vi "TDMS Timestamp and Data Double.vi"(6 "channel name(s) in (Untitled)":string[](array[string]), 7 "timestamp":timestamp, 8 "error in (no error)":errorcluster, 9 "group name in (Untitled)":string, 10 "Array":dbl[](array[numeric]), 11 "Refnum in":refnum<k34>) -> (0 "error out":errorcluster, 3 "Refnum out":refnum<k34>)   [LabVIEW 2014]
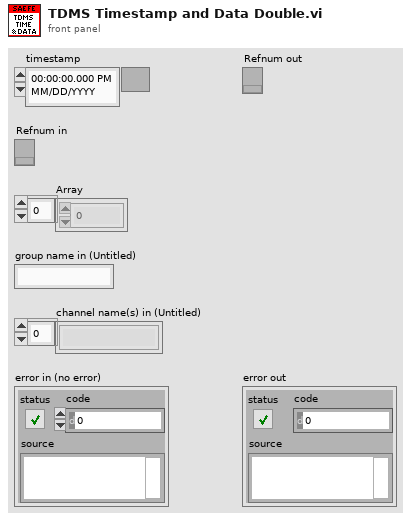
[diagram p1: front panel]
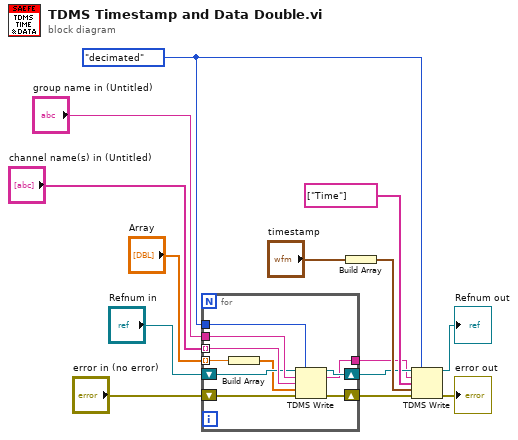
[diagram p0: block diagram]
diagram:
  w12 = enum16{"decimated", "interleaved"}."decimated" ("data layout (0:decimated)")
  n1 = for {
    tunnel: w12 -> [w24]
    tunnel: "Array" -> [w17] mode=indexing
    tunnel: "channel name(s) in (Untitled)" -> [w21] mode=indexing
    tunnel: "group name in (Untitled)" -> [w20]
    shift-right: [w23] -> w7
    shift-left: "error in (no error)" -> [w19]
    shift-right: [w22] -> w6
    shift-left: "Refnum in" -> [w18]
    tunnel: [w15] -> w1
    n2 = Build Array(w17) -> (w16:dbl[])
    n3 = TDMS Write(0:w18, 1:w24, 5:w20, 7:w21, 9:w16, 11:w19) -> (4:w22:refnum<k34>, 6:w15:string, 15:w23:errorcluster)  [unwired: 1 out]
  }
  n4 = Build Array("timestamp") -> (w14:timestamp[])
  n5 = TDMS Write(0:w6, 1:w12, 5:w1, 7:string[] ["Time"] ("channel name(s) in (Untitled)"), 9:w14, 11:w7) -> (4:→"Refnum out":refnum<k34>, 15:→"error out":errorcluster)  [unwired: 2 out]
